vi "SendProgramInitial.vi"(8 "error in (no error)":errorcluster, 11 "Queue in":refnum<queue>) -> (0 "error out":errorcluster, 3 "Queue out":refnum<queue>)   [LabVIEW 2014, in "ProgramInitial.lvclass"]
uses:
  ProgramInitial.lvclass
  AbstractionMessage/AbstractionMessage.lvclass
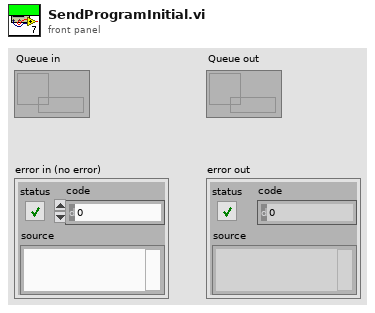
[diagram p1: front panel]
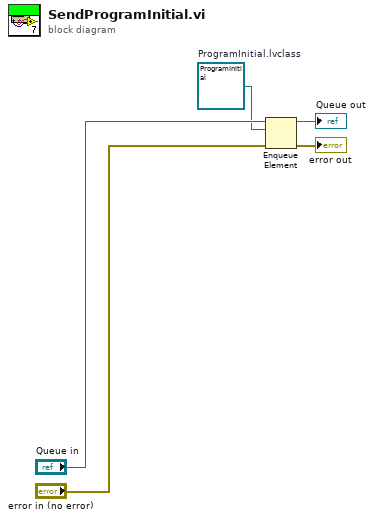
[diagram p0: block diagram]
diagram:
  w1 = refnum<class "ProgramInitial.lvclass"> refnum  # ProgramInitial.lvclass
  n1 = Enqueue Element(queue="Queue in", element=w1, error in (no error)="error in (no error)") -> (queue out=→"Queue out":refnum<queue>, error out=→"error out":errorcluster)  [unwired: 1 in, 1 out]
